vi "LVClass_CorrectionDataManager SetWaveFrontCorrectorPreferences.vi"(0 "CorrectionDataManager in":refnum<class "CorrectionDataManager.lvclass">, 9 "Wavefront Corrector State":T1[](array[typedef]), 11 "error in (no error)":errorcluster) -> (4 "CorrectionDataManager out":refnum<class "CorrectionDataManager.lvclass">, 8 "New data needed":bool, 15 "error out":errorcluster)   [LabVIEW 2020, in "CorrectionDataManager.lvclass"]
doc: "Wavefront corrector actuators preferences setter. .\n\n<B>corrdata_managerIn</B> : CorrDataManager object.\n<B>corrdata_managerOut</B> : CorrDataManager object.\n<B>min</B> : WavefrontCorrector preferences : lowest command value.\n<B>max</B> : WavefrontCorrector preferences : highest command value.\n<B>validity</B> : WavefrontCorrector preferences : status.\n<B>fixed_value</B> : WavefrontCorrector preferences : fixed positions.\n<B>new_data_needed</B> : if true, indicates that interaction matrix has been erased."
uses:
  CorrectionDataManager.lvclass
  Wavefront Corrector states - ONE.ctl
  CorrectionDataManager.lvclass/CorrectionDataManager.ctl
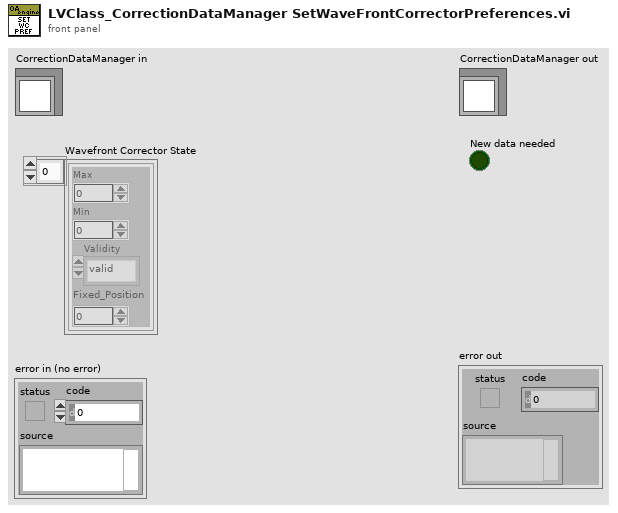
[diagram p1: front panel]
types:
  T1 = typedef "Wavefront Corrector states - ONE.ctl" = cluster{"Max":sgl, "Min":sgl, "Validity":enum16{"valid", "fixed", "invalid"}, "Fixed_Position":sgl}
  T2 = typedef "ClassID.ctl" = i64
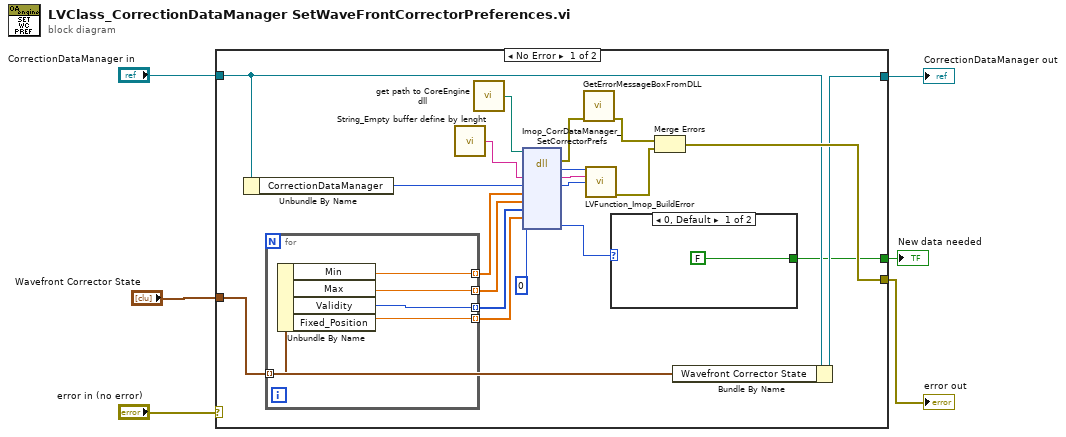
[diagram p0: block diagram]
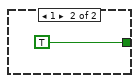
[diagram p2: hidden frame]
diagram:
  n1 = case shown="No Error" "error in (no error)" {
    selector: "error in (no error)" -> [_ w35]
    tunnel: [w24 w35] -> w3
    tunnel: [w12 w34] -> w4
    tunnel: "CorrectionDataManager in" -> [w13 w34]
    tunnel: "Wavefront Corrector State" -> [w11 _]
    tunnel: [w8 _] -> w1
    frame No Error {
      n2 = Unbundle By Name(w13) -> ("CorrectionDataManager"=w14:T2)
      n3 = for {
        tunnel: w11 -> [w33] mode=indexing
        tunnel: [w32] -> w16 mode=indexing
        tunnel: [w31] -> w15 mode=indexing
        tunnel: [w30] -> w18 mode=indexing
        tunnel: [w29] -> w17 mode=indexing
        n4 = Unbundle By Name(w33) -> ("Min"=w32:sgl, "Max"=w31:sgl, "Validity"=w30:enum16{"valid", "fixed", "invalid"}, "Fixed_Position"=w29:sgl)
      }
      n5 = call "String_Empty buffer define by lenght.vi"() -> ("Empty buffer"=w22:string)  [unwired: 1 in]
      n6 = call "get path to CoreEngine dll.vi"() -> ("path to wavekit library"=w23:path)  [unwired: 14 in, 1 out]
      n7 = dll-call lib="D:/soft/HASO_v3/SVN_trunk/ImOpCoreEngine4_LV2011/DLLs/c_interface_vc100.dll" fn="Imop_CorrDataManager_SetCorrectorPrefs"(path in=w23, "message"=w22, "CorrDataManager"=w14, "min"=w16, "max"=w15, "validity"=w18, "fixed_value"=w17, "New data needed"=u8 0) -> (error out=w21:errorcluster, "return type"=w20:i32, "message"=w19:string, "CorrDataManager"=w7:i64, "New data needed"=w9:u8)  [unwired: 6 in, 1 out]
      n8 = call "GetErrorMessageBoxFromDLL.vi"("error IN"=w21) -> ("error OUT"=w26:errorcluster)  [unwired: 10 in]
      n9 = call "LVFunction_Imop_BuildError.vi"("code"=w20, "String to Prepend to source (\"\")"=w19, "Adresse"=w7) -> ("error out"=w25:errorcluster)  [unwired: 12 in]
      n10 = case shown="0, Default" w9 {
        tunnel: [FALSE TRUE] -> w8
        frame 0, Default {
        }
        frame 1 {
        }
      }
      n11 = Merge Errors(w26, w25) -> (w24:errorcluster)
      n12 = Bundle By Name(cluster=w13, "Wavefront Corrector State"=w11) -> (w12:refnum<class "CorrectionDataManager.lvclass">)
    }
    frame Error {
    }
  }
  "error out" <- w3
  "CorrectionDataManager out" <- w4
  "New data needed" <- w1
